vi "average-2Darray-SD_int.vi"(1 "2D array":i32[][](array[numeric])) -> (0 "out array":dbl[](array[numeric]))   [LabVIEW 2015]
uses:
  <vilib>/Analysis/baseanly.llb/Mean (DBL).vi
  <vilib>/Analysis/NI_AALBase.lvlib
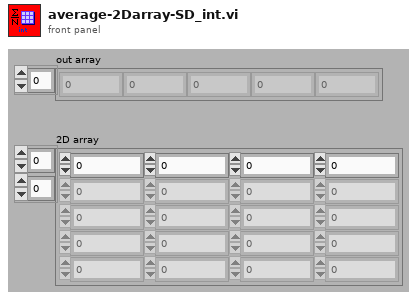
[diagram p1: front panel]
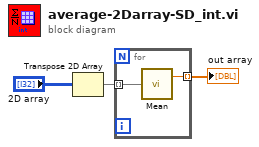
[diagram p0: block diagram]
diagram:
  n1 = Transpose 2D Array(2D array="2D array") -> (transposed array=w3:i32[][])
  n2 = for {
    tunnel: w3 -> [w5] mode=indexing
    tunnel: [w4] -> w1 mode=indexing
    n3 = call-poly <vilib>:"Mean.vi"("X"=w5) -> ("mean"=w4:dbl)  [unwired: 1 out]
  }
  "out array" <- w1
